vi "TCP_Test No Connection Errors.vi"(8 "error in":errorcluster) -> (0 "error out":errorcluster)   [LabVIEW 2013]
uses:
  <vilib>/addons/_JKI Toolkits/Caraya/classes/Assert/Assert Equal Value_Variant.vi
  <vilib>/LabVIEW Open Source Project/MQTT Connection/MQTT_Connection/Connection/Connection.lvclass
  source/MQTT_TCP/Connection/TCPConnection.lvclass
  <vilib>/addons/_JKI Toolkits/Caraya/classes/Test/Test.lvclass
  <vilib>/addons/_JKI Toolkits/Caraya/classes/Assert/Assert.lvclass
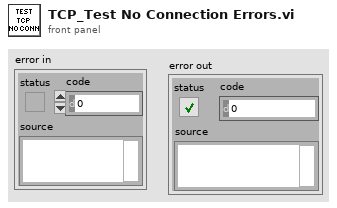
[diagram p1: front panel]
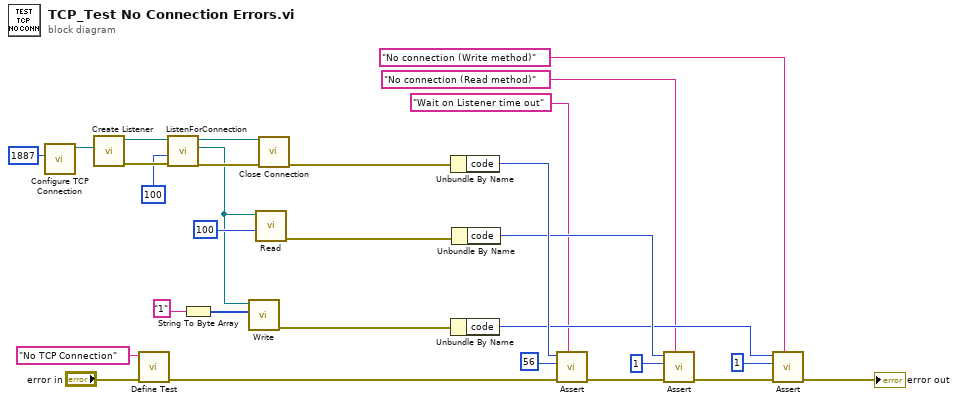
[diagram p0: block diagram]
diagram:
  n1 = call "Configure TCP Connection.vi"("remote port (80)"=u16 1887 ("port")) -> ("TCPConnection"=w20:refnum<class "TCPConnection.lvclass">)  [unwired: 9 in, 1 out]
  n2 = call <vilib>:"Create Listener.vi"("Connection Configuration"=w20) -> ("error out"=w26:errorcluster, "Listener"=w29:refnum<class "Connection.lvclass">)  [unwired: 9 in]
  n3 = call <vilib>:"Define Test.vi"("error in (no error)"="error in", "Label (VI Title)"="No TCP Connection") -> ("error out"=w14:errorcluster)  [unwired: 9 in]
  n4 = call <vilib>:"ListenForConnection.vi"("error in (no error)"=w26, "timeout (2000 ms)"=100 ("timeout ms (wait forever: -1)"), "Listener"=w29) -> ("error out"=w27:errorcluster, "Connection"=w21:refnum<class "Connection.lvclass">, "Listener out"=w28:refnum<class "Connection.lvclass">)  [unwired: 5 in, 1 out]
  n5 = String To Byte Array(string="1" ("data in")) -> (unsigned byte array=w24:u8[])
  n6 = call <vilib>:"Write.vi"("Bytes"=w24, "Connection in"=w21) -> ("error out"=w17:errorcluster)  [unwired: 8 in, 1 out]
  n7 = call <vilib>:"Read.vi"("timeout (2000 ms)"=100 ("bytes to read"), "TCPConnection in"=w21) -> ("error out"=w16:errorcluster)  [unwired: 5 in, 4 out]
  n8 = call <vilib>:"Close Connection.vi"("error in (no error)"=w27, "Connection in"=w28) -> ("error out"=w18:errorcluster)  [unwired: 8 in, 1 out]
  n9 = Unbundle By Name(w18) -> ("code"=w13:i32)
  n10 = Unbundle By Name(w17) -> ("code"=w8:i32)
  n11 = Unbundle By Name(w16) -> ("code"=w9:i32)
  n12 = call-poly <vilib>:"Assert.vi"("Label"="Wait on Listener time out" ("Label (VI Title)"), "error in (no error)"=w14, "Y"=56 ("code"), "X"=w13) -> ("error out"=w11:errorcluster)  [unwired: 7 in]
  n13 = call-poly <vilib>:"Assert.vi"("Label"="No connection (Read method)" ("Label (VI Title)"), "error in (no error)"=w11, "Y"=1 ("code"), "X"=w9) -> ("error out"=w10:errorcluster)  [unwired: 7 in]
  n14 = call-poly <vilib>:"Assert.vi"("Label"="No connection (Write method)" ("Label (VI Title)"), "error in (no error)"=w10, "Y"=1 ("code"), "X"=w8) -> ("error out"=→"error out":errorcluster)  [unwired: 7 in]
